vi "motor control develop.vi"() -> ()   [LabVIEW 2016]
panel:
  out "MicroStrain (ue), (AI 3)":dbl
  in  "Load limit lower (N)":dbl=-1000.0 min=-4500.0 max=4500.0 step=10.0
  in  "Load limit upper (N)":dbl=1000.0 min=-4500.0 max=4500.0 step=10.0
  in  "Displacement limit lower (mm)":dbl=-3.0 min=-100000.0 max=10.0 step=0.1
  in  "Displacement limit upper (mm)":dbl=3.0 min=-10.0 max=100000.0 step=0.1
  in  "Select a file to save":path=path "C:/Users/ZheChen/Desktop/UMich work/Labview for Tensile Stage/measurement.lvm" caption="Filename"
  out "Present Text":string
  out "Elapsed Time Text":string
  in  "Update File":bool
  out "Signal vs time chart":dynamicdata(graph)
  out "Displacement-Load Graph":cluster{"Y":dbl[], "Y":dbl[]}[](graph)
  in  "Samples per second to record":i32=1 min=1 max=100 step=1
  out "Load (N), (AI 0)":dbl format="%4.1f"
  out "Displacement (mm), (AI 1)":dbl format="%4.3f"
  out "Loop":dbl
  in  "stop":bool
  in  "Tension/Compression (P0.1)":bool
  in  "Motor On/Off (P0.0)":bool
  in  "Select Device":tag="Dev3_simulated"
  in  "Moter Speed (um/s)":dbl=0.5 min=0.0 max=20.0 step=0.1
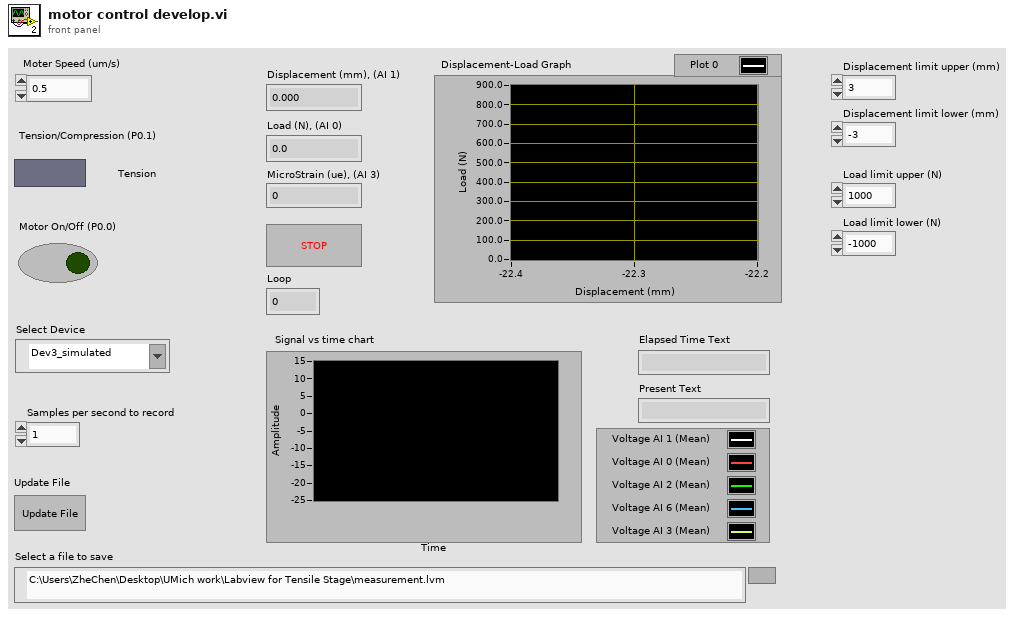
[diagram p1: front panel]
types:
  T1 = typedef "NI_Matrix.lvlib/RealMatrix.ctl" = dbl[][]
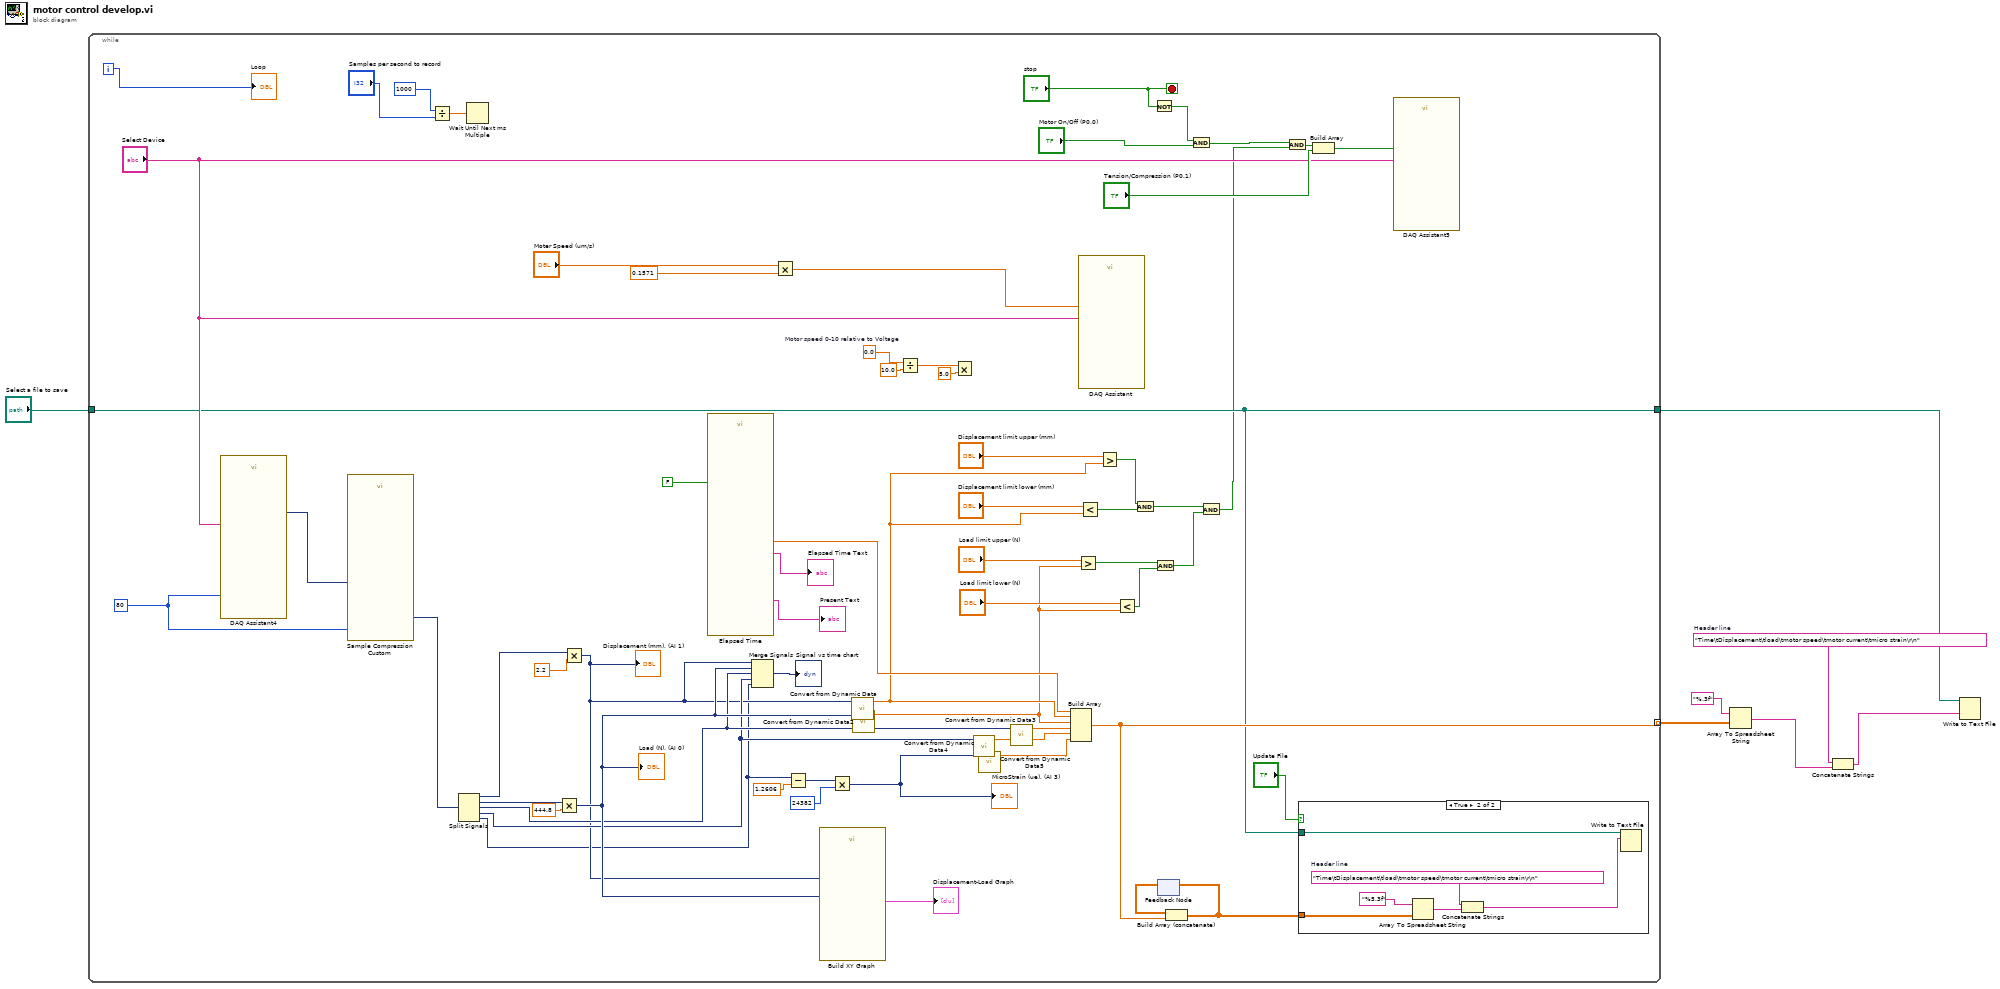
[diagram p0: block diagram]
diagram:
  w5 = "Time\tDisplacement\tload\tmotor speed\tmotor current\tmicro strain\r\n"  # Header line
  n1 = while {
    tunnel: [w34] -> w7
    tunnel: [w49] -> w2 mode=indexing
    tunnel: "Select a file to save" -> [w34]
    i -> [w59]
    stop <- "stop" stop-if-true
    w33 = 0.0  # Motor speed 0-10 relative to Voltage
    w37 = u32 80 ("Size")
    n2 = call "DAQ Assistant4"("number of samples"=w37, "device name"="Select Device") -> ("data"=w39:dynamicdata)  [unwired: 15 in, 2 out]
    n3 = call "Sample Compression Custom.vi"("Size"=w37, "Signals"=w39) -> ("Mean"=w38:dynamicdata)  [unwired: 7 in, 2 out]
    n4 = Divide(x=u32 1000 ("millisecond multiple"), y="Samples per second to record") -> (x/y=w53:dbl)
    n5 = Split Signals(w38) -> (w66:dynamicdata, w67:dynamicdata, w44:dynamicdata, w43:dynamicdata, w13:dynamicdata)  [unwired: 5 in]
    n6 = Wait Until Next ms Multiple(millisecond multiple=w53) -> ()  [unwired: 1 out]
    n7 = Multiply(x=w67, y=444.8) -> (x*y=w52:dynamicdata)
    "Load (N), (AI 0)" <- w52
    n8 = Multiply(x=w66, y=2.2) -> (x*y=w27:dynamicdata)
    "Displacement (mm), (AI 1)" <- w27
    n9 = call "Elapsed Time"("Auto Reset"=FALSE ("Reset")) -> ("Present Text"=→"Present Text":string, "Elapsed Time (s)"=w50:dbl, "Elapsed Time Text"=→"Elapsed Time Text":string)  [unwired: 11 in, 5 out]
    n10 = Merge Signals(w27, w52, w44, w43, w13) -> (→"Signal vs time chart":dynamicdata)
    n11 = Multiply(x="Moter Speed (um/s)", y=0.1571) -> (x*y=w30:dbl)
    n12 = Subtract(x=w13, y=1.2606) -> (x-y=w11:dynamicdata)
    n13 = call "Build XY Graph"("Y Input"=w52, "X Input"=w27) -> ("XY Graph"=→"Displacement-Load Graph":cluster{"X":dbl[], "Y":dbl[]}[])  [unwired: 8 in, 1 out]
    n14 = Multiply(x=w11, y=24382) -> (x*y=w9:dynamicdata)
    "MicroStrain (ue), (AI 3)" <- w9
    n15 = call "Convert from Dynamic Data"("Dynamic Data Type"=w27) -> ("Scalar"=w26:dbl)  [unwired: 3 in]
    n16 = call "Convert from Dynamic Data2"("Dynamic Data Type"=w52) -> ("Scalar"=w23:dbl)  [unwired: 3 in]
    n17 = Divide(x=w33, y=10.0) -> (x/y=w60:dbl)
    n18 = Multiply(x=w60, y=5.0) -> ()  [unwired: 1 out]
    n19 = call "Convert from Dynamic Data4"("Dynamic Data Type"=w43) -> ("Scalar"=w45:dbl)  [unwired: 3 in]
    n20 = call "Convert from Dynamic Data5"("Dynamic Data Type"=w9) -> ("Scalar"=w14:dbl)  [unwired: 3 in]
    n21 = call "Convert from Dynamic Data3"("Dynamic Data Type"=w44) -> ("Scalar"=w46:dbl)  [unwired: 3 in]
    n22 = Build Array(w50, w26, w23, w46, w45, w14) -> (w49:dbl[])
    n23 = Greater?(x="Load limit upper (N)", y=w23) -> (0:w20:bool)
    n24 = call "DAQ Assistant"("data"=w30, "device name"="Select Device") -> ()  [unwired: 16 in, 2 out]
    n25 = Less?(x="Displacement limit lower (mm)", y=w26) -> (x < y?=w21:bool)
    n26 = Greater?(x="Displacement limit upper (mm)", y=w26) -> (0:w22:bool)
    n27 = Less?(x="Load limit lower (N)", y=w23) -> (x < y?=w19:bool)
    n28 = And(x=w22, y=w21) -> (x .and. y?=w18:bool)
    n29 = Not(x="stop") -> (.not. x?=w40:bool)
    n30 = And(x=w20, y=w19) -> (x .and. y?=w17:bool)
    n31 = feedback #1() -> (w48:T1)  [unwired: 1 in]
    n32 = Build Array (concatenate)(w48, w49) -> (w47:T1)
    n33 = feedback-in #1(w47) -> ()
    n34 = And(x=w40, y="Motor On/Off (P0.0)") -> (x .and. y?=w16:bool)
    n35 = And(x=w18, y=w17) -> (x .and. y?=w8:bool)
    n36 = And(x=w16, y=w8) -> (x .and. y?=w15:bool)
    n37 = case shown="True" "Update File" {
      tunnel: w34 -> [_ w75]
      tunnel: w47 -> [_ w70]
      frame False {
      }
      frame True {
        w73 = "Time\tDisplacement\tload\tmotor speed\tmotor current\tmicro strain\r\n"  # Header line
        n38 = Array To Spreadsheet String(array=w70, 3:"%5.3f") -> (spreadsheet string=w72:string)  [unwired: 1 in]
        n39 = Concatenate Strings(w73, w72) -> (w71:string)
        n40 = Write to Text File(file (use dialog)=w75, text=w71) -> ()  [unwired: 2 in, 3 out]
      }
    }
    n41 = Build Array(w15, "Tension/Compression (P0.1)") -> (w64:bool[])
    n42 = call "DAQ Assistant5"("data"=w64, "device name"="Select Device") -> ()  [unwired: 16 in, 2 out]
    "Loop" <- w59
  }
  n43 = Array To Spreadsheet String(array=w2, 3:"%.3f") -> (spreadsheet string=w4:string)  [unwired: 1 in]
  n44 = Concatenate Strings(w5, w4) -> (w3:string)
  n45 = Write to Text File(file (use dialog)=w7, text=w3) -> ()  [unwired: 2 in, 3 out]
